vi "fpga_LineInputs-Bank3-0.vi"() -> (0 "DataLines":T1)   [LabVIEW 2011]
uses:
  <vilib>/rvi/eio/common/nirviEmuTemplateMethod_errors.vi
  <vilib>/eio/EIONode/EIONode.xnode
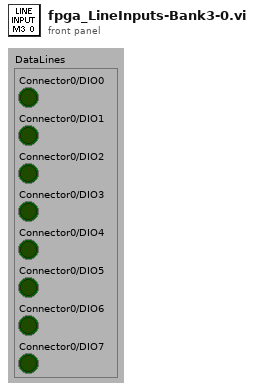
[diagram p1: front panel]
types:
  T1 = cluster{"Connector0/DIO0":bool, "Connector0/DIO1":bool, "Connector0/DIO2":bool, "Connector0/DIO3":bool, "Connector0/DIO4":bool, "Connector0/DIO5":bool, "Connector0/DIO6":bool, "Connector0/DIO7":bool}
  T2 = cluster{"Connector3/DIO17":bool, "Connector0/DIO18":bool, "Connector3/DIO15":bool, "Connector0/DIO20":bool, "Connector3/DIO37":bool, "Connector0/DIO24":bool, "Connector3/DIO27":bool, "Connector3/DIO28":bool}
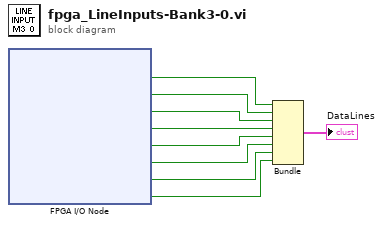
[diagram p0: block diagram]
diagram:
  n1 = xnode "FPGA I/O Node"() -> ("Connector3/DIO17"=w9:bool, "Connector0/DIO18"=w8:bool, "Connector3/DIO15"=w7:bool, "Connector0/DIO20"=w6:bool, "Connector3/DIO37"=w5:bool, "Connector0/DIO24"=w4:bool, "Connector3/DIO27"=w3:bool, "Connector3/DIO28"=w2:bool)  [unwired: 8 in, 8 out]
  n2 = Bundle("Connector3/DIO17"=w9, "Connector0/DIO18"=w8, "Connector3/DIO15"=w7, "Connector0/DIO20"=w6, "Connector3/DIO37"=w5, "Connector0/DIO24"=w4, "Connector3/DIO27"=w3, "Connector3/DIO28"=w2) -> (→"DataLines":T2)  [unwired: 1 in]
